vi "DAQ2.vi"(1 "sampling info":cluster{"Fs":dbl, "#s":dbl}={"Fs"=1001.0, "#s"=1000.0}) -> (0 "Waveform":waveform(dbl)={"t0"=timestamp(50.94905094905095 s since 1904-01-01), "dt"=0.000999000999000999, "Y"=array[1000 elements]})   [LabVIEW 2018]
uses:
  <vilib>/measure/NI_MABase.lvlib
panel:
  in  "offset":dbl format="%0.2p"
  in  "phase":dbl format="%.2p"
  in  "rumore":dbl=0.02000000000000001 min=0.0 step=0.01 format="%.2p"
  in  "signal type":T1(ring)
  in  "amplitude":dbl=2.0 format="%0.2p"
  in  "frequency":dbl=50.0 min=0.0 step=0.5 format="%0.2p"
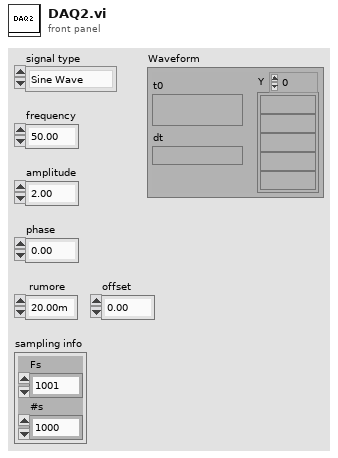
[diagram p1: front panel]
types:
  T1 = enum16{"Sine Wave", "Triangle Wave", "Square Wave", "Sawtooth Wave"}
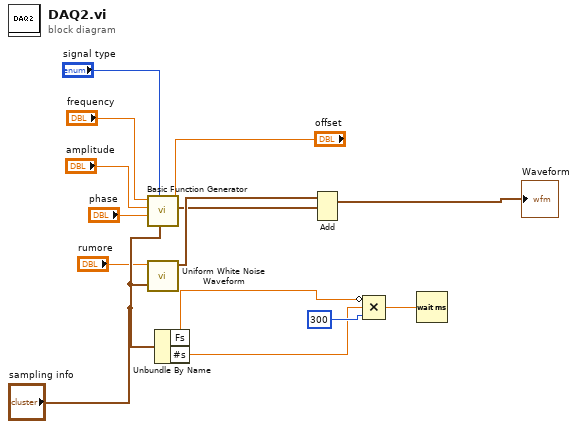
[diagram p0: block diagram]
diagram:
  n1 = call <vilib>:"Basic Function Generator.vi"("offset"="offset", "sampling info"="sampling info", "signal type"="signal type", "phase"="phase", "amplitude"="amplitude", "frequency"="frequency") -> ("signal out"=w11:waveform(dbl))  [unwired: 3 in, 2 out]
  n2 = call <vilib>:"Uniform White Noise Waveform.vi"("sampling info"="sampling info", "amplitude"="rumore") -> ("signal out"=w12:waveform(dbl))  [unwired: 8 in, 1 out]
  n3 = Unbundle By Name("sampling info") -> ("Fs"=w6:dbl, "#s"=w7:dbl)
  n4 = Add(1:w11, 2:w12) -> (0:→"Waveform":waveform(dbl))  [unwired: 1 in, 1 out]
  n5 = Compound Arithmetic op=MULTIPLY(invert w6, w7, u32 300 ("millisecond timer value")) -> (w9:dbl)
  n6 = Wait (ms)(milliseconds to wait=w9) -> ()  [unwired: 1 out]
